vi "Pre Launch Init.vi"(11 "CS++BaseActor in":refnum<class "CS++BaseActor.lvclass">) -> (0 "error out":errorcluster, 3 "CS++BaseActor out":refnum<class "CS++BaseActor.lvclass">)   [LabVIEW 2015, in "CS++BaseActor.lvlib" / "CS++BaseActor.lvclass"]
doc: "(<B>Filename</B>: Actor Framework.lvlib:Actor.lvclass:Pre Launch Init.vi)\n\nDefines behavior that occurs after the Launch Actor method is invoked but before the actor's Actor Core method begins running.\n\nThe Pre Launch Init method is guaranteed to finish before the Launch Actor method returns to its caller and before the actor itself receives any messages. Any references that the Pre Launch Init method obtains are guaranteed to have the same lifetime as the actor itself. Any errors that the Pre Launch Init method returns will abort the launch.\n\nBy default, this method does nothing. A descendant class may override it to define behavior."
uses:
  CS++BaseActor.lvclass
  Libraries/Base/FGV Action.ctl
  CS++BaseActor.lvclass/CS++BaseActor.ctl
  Libraries/Base/Severity.ctl
  <vilib>/ActorFramework/Actor/Actor.lvclass
  Libraries/Base/CS++Base.lvlib
  Libraries/Utilities/CS++Utilities.lvlib
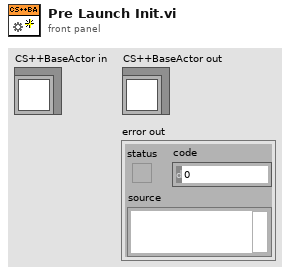
[diagram p1: front panel]
types:
  T1 = typedef "CS++Base.lvlib/FGV Action.ctl" = enum16{"add", "replace", "read", "remove", "reset", "get attributes"}
  T2 = typedef "CS++Base.lvlib/Severity.ctl" = enum16{"emergency", "alert", "critical", "error", "warning", "notice", "info", "debug"}
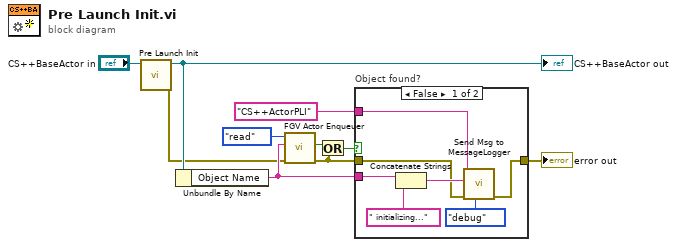
[diagram p0: block diagram]
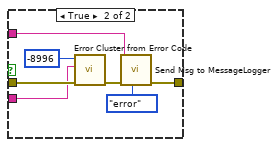
[diagram p2: hidden frame]
diagram:
  n1 = call-parent "Pre Launch Init.vi"("Actor in"="CS++BaseActor in") -> ("error out"=w5:errorcluster, "Actor out"=w7:refnum<class "CS++BaseActor.lvclass">)  [unwired: 9 in]
  "CS++BaseActor out" <- w7
  n2 = Unbundle By Name(w7) -> ("Object Name"=w6:string)
  n3 = call "FGV Actor Enqueuer.vi"("Error In"=w5, "Actor Name"=w6, "Action (read)"=FGV_Action."read") -> ("Error Out"=w1:errorcluster, "Success"=w2:bool)  [unwired: 4 in, 3 out]
  n4 = Or(x=w2, y=w1) -> (x .or. y?=w3:bool)
  n5 = case "Object found?" shown="False" w3 {
    tunnel: [w16 w24] -> w9
    tunnel: w6 -> [w13 w20]
    tunnel: w1 -> [w11 w22]
    tunnel: "CS++ActorPLI" ("Message Tag") -> [w12 w18]
    frame False {
      n6 = Concatenate Strings(w13, " initializing..." ("string")) -> (w15:string)
      n7 = call "Send Msg to MessageLogger.vi"("Severity Code (info)"=Severity."debug", "Error In"=w11, "Message Content"=w15, "Message Tag"=w12) -> ("Error Out"=w16:errorcluster)  [unwired: 7 in]
    }
    frame True {
      n8 = call "Error Cluster from Error Code.vi"("Error In"=w22, "Error Message (\"\")"=w20, "Error Code (0)"=-8996 ("error code (0)")) -> ("Error Out"=w19:errorcluster)  [unwired: 8 in]
      n9 = call "Send Msg to MessageLogger.vi"("Severity Code (info)"=Severity."error", "Error In"=w19, "Message Tag"=w18) -> ("Error Out"=w24:errorcluster)  [unwired: 8 in]
    }
  }
  "error out" <- w9
